vi "DeppGetRegSet.vi"(7 "Overlap?":bool, 8 "Error In":errorcluster, 10 "Addresses":u8[](array[numeric]), 11 "Device Handle":u32) -> (0 "Error Out":errorcluster, 2 "Data":u8[](array[numeric]), 3 "Device Handle":u32)   [LabVIEW 2011, in "LVH-Adept.lvlib" / "DEPP.lvlib"]
uses:
  DEPP.lvlib
  Private/Type Defs/Error.ctl
  depp.dll
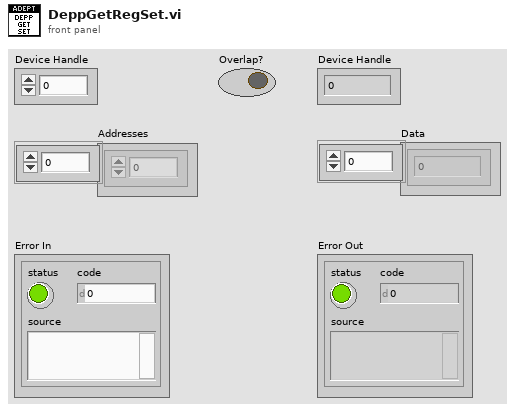
[diagram p1: front panel]
types:
  T1 = typedef "LVH-Adept.lvlib/DEPP.lvlib/Error.ctl" = enum16{"Unknown", "Enable", "Enable Port", "Get Register", "Get Register Repeat", "Get Register Set", "Put Register", "Put Register Repeat", "Put Register Set", "Disable", "Set Pair Size"}
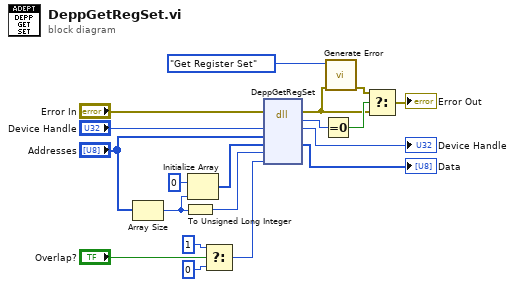
[diagram p0: block diagram]
diagram:
  n1 = Array Size(array="Addresses") -> (size(s)=w2:i32)
  n2 = To Unsigned Long Integer(number=w2) -> (unsigned 32bit integer=w1:u32)
  n3 = Initialize Array(u8 0 ("t"), w2) -> (w5:u8[])
  n4 = Select(t=u8 1, s="Overlap?", f=u8 0) -> (s? t:f=w7:u8)
  n5 = dll-call lib="depp.dll" fn="DeppGetRegSet"(error in="Error In", "hif"="Device Handle", "pbAddr"="Addresses", "pbData"=w5, "cbData"=w1, "fOverlap"=w7) -> (error out=w11:errorcluster, "Success"=w18:u32, "hif"=→"Device Handle":u32, "pbData"=→"Data":u8[])  [unwired: 5 in, 1 out]
  n6 = Equal To 0?(x=w18) -> (x = 0?=w17:bool)
  n7 = call "Generate Error.vi"("Error In"=w11, "DEPP Error"=Error."Get Register Set") -> ("Error Out"=w12:errorcluster)  [unwired: 9 in]
  n8 = Select(t=w12, s=w17, f=w11) -> (s? t:f=→"Error Out":errorcluster)
